vi "Get Error State.vi"(11 "error in (no error)":errorcluster) -> (8 "Error state":string[][](array[string]), 14 "updated":bool, 15 "error out":errorcluster)   [LabVIEW 2011]
uses:
  E&S/Monitor/Actino S&E monitor.ctl
  E&S/String outpyt type.ctl
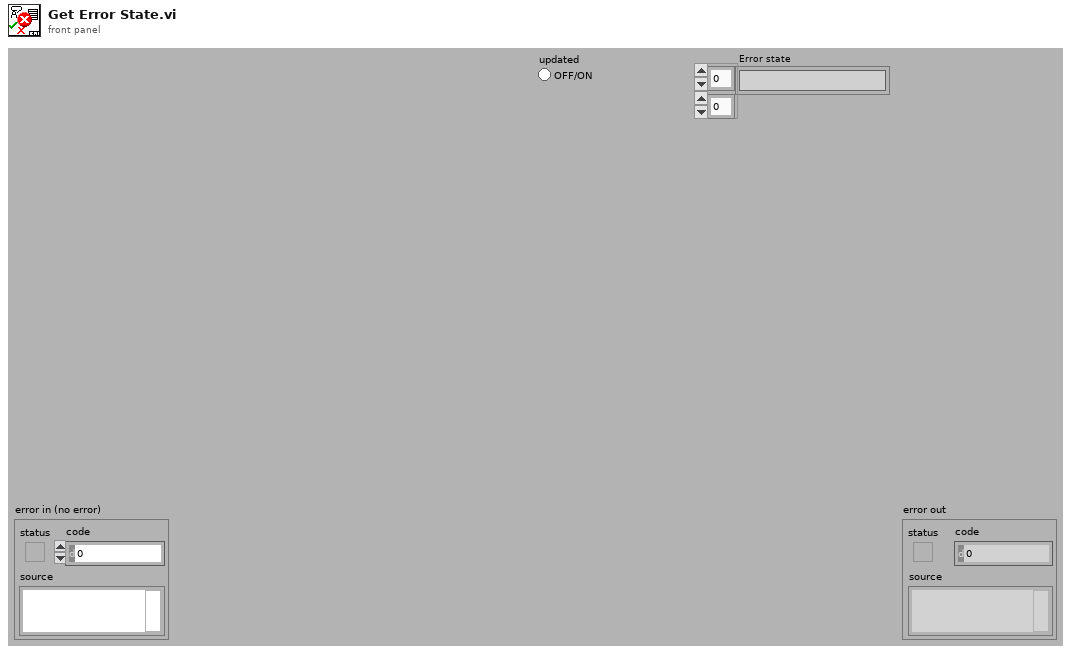
[diagram p1: front panel]
types:
  T1 = typedef "Actino S&E monitor.ctl" = enum16{"GET(type history)", "SET S&E", "(Re)Init", "Get Error state", "Get  Alarm state", "Get All", "Get last  250", "Get Alarm History"}
  T2 = typedef "_emi_ S&E Message.ctl" = cluster{"Type":T3, "Originate time":dbl, "System":u8, "Loop":u16, "Sub ID":u16, "Elevated priority":bool, "E&S Message content":variant}
  T3 = typedef "_emi_ S&E Message type.ctl" = enum16{"Error/Warning", "Note", "Debug", "Event", "Alarm Analog", "Alarm Digital", "Annotation"}
  T4 = typedef "String outpyt type.ctl" = enum16{"Full File hist", "Simple File hist", "Displ Hist one type", "Displ Hist mult types", "Displ Stat one type", "Displ Stat Mult type"}
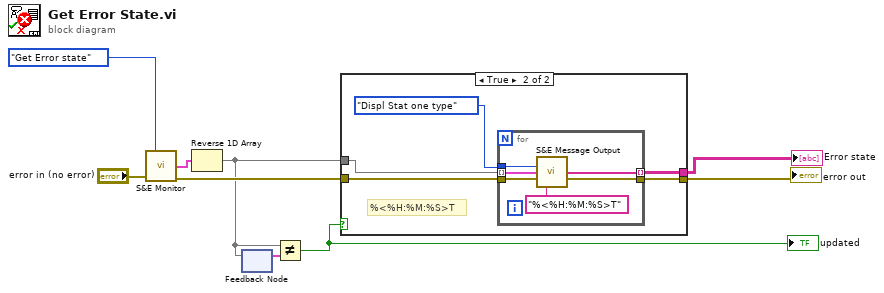
[diagram p0: block diagram]
diagram:
  n1 = call "S&E Monitor.vi"("Action(GET 250)"=Actino_S&E_monitor."Get Error state", "error in (no error)"="error in (no error)") -> ("S&E"=w7:T2[], "error out"=w4:errorcluster)  [unwired: 12 in]
  n2 = Reverse 1D Array(array=w7) -> (reversed array=w3:T2[])
  n3 = feedback-in #1(w3) -> ()
  n4 = feedback #1() -> (w6:T2[])  [unwired: 1 in]
  n5 = Not Equal?(x=w3, y=w6) -> (x != y?=w5:bool)
  "updated" <- w5
  n6 = case shown="True" w5 {
    tunnel: w4 -> [w10 w14]
    tunnel: w3 -> [_ w13]
    tunnel: [w10 w12] -> w1
    tunnel: [_ w11] -> w2
    frame False {
    }
    frame True {
      # "%<%H:%M:%S>T"
      n7 = for {
        tunnel: String_outpyt_type."Displ Stat one type" ("Type(File Hist)") -> [w21]
        tunnel: w14 -> [w20]
        tunnel: w13 -> [w19] mode=indexing
        tunnel: [w18] -> w12
        tunnel: [w16] -> w11 mode=indexing
        n8 = call "S&E Message Output.vi"("Type(File Hist)"=w21, "E&S Message"=w19, "error in (no error)"=w20, "Time format(%T)"="%<%H:%M:%S>T") -> ("Array of strings"=w16:string[], "error out"=w18:errorcluster)  [unwired: 9 in, 1 out]
      }
    }
  }
  "error out" <- w1
  "Error state" <- w2
